vi "Error classifier.vi"(11 "Error in":errorcluster) -> (4 "Classified Ouput Error":T1, 15 "Error out":errorcluster)   [LabVIEW 2020, in "PSRR Monitor.lvlib"]
doc: "This VI is used to classify the error which is generated by the PSRR meter and will give the classified error to the main PSRR module."
uses:
  PSRR Monitor.lvlib
  Typedefs/Error Details.ctl
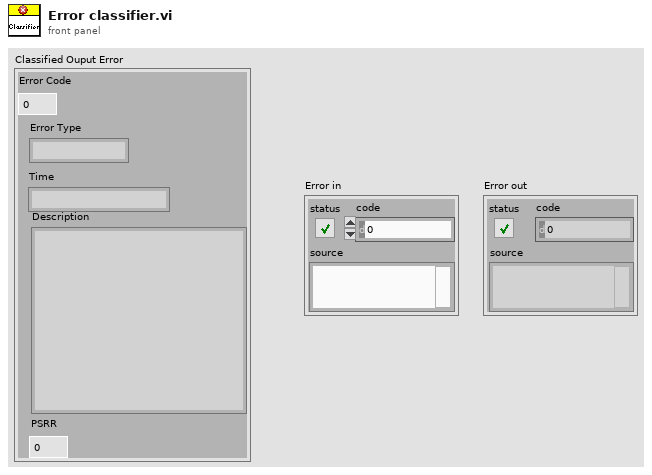
[diagram p1: front panel]
types:
  T1 = typedef "Error Details.ctl" = cluster{"Error Code":i32, "Error Type":string, "Time":string, "Description":string, "PSRR":i32}
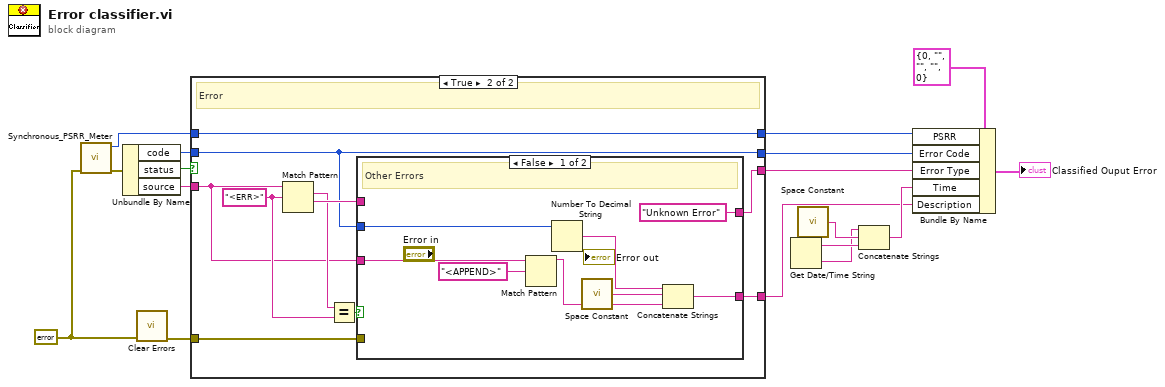
[diagram p0: block diagram]
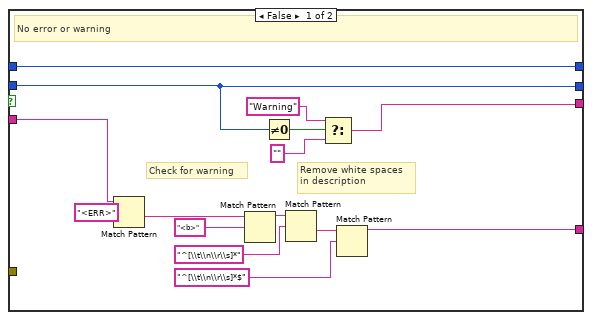
[diagram p2: hidden frame]
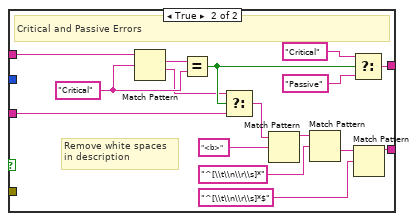
[diagram p3: hidden frame]
diagram:
  w2 = errorcluster {"status"=FALSE, "code"=0, "source"=""} ("error in")
  n1 = call "Synchronous_PSRR_Meter.vi"("error in"=w2) -> ("error out"=w17:errorcluster, "PSRR (dB)"=w4:i32)  [unwired: 9 in]
  n2 = Unbundle By Name(w17) -> ("code"=w14:i32, "status"=w15:bool, "source"=w16:string)
  n3 = call <vilib>:"Clear Errors.vi"("error in (no error)"=w2) -> ("error out"=w1:errorcluster)  [unwired: 5 in, 1 out]
  n4 = case shown="True" w15 {
    tunnel: w16 -> [w26 w36]
    tunnel: w14 -> [w29 w35]
    tunnel: [w29 w35] -> w12
    tunnel: [w28 w42] -> w11
    tunnel: [w19 w40] -> w5
    tunnel: w4 -> [w18 w34]
    tunnel: [w18 w34] -> w3
    tunnel: w1 -> [_ w33]
    frame False {
      # "Check for warning"
      # "Remove white spaces\nin description"
      # "No error or warning"
      n5 = Match Pattern(string=w26, regular expression="<ERR>") -> (after substring=w20:string)  [unwired: 1 in, 3 out]
      n6 = Match Pattern(string=w20, regular expression="<b>") -> (before substring=w21:string)  [unwired: 1 in, 3 out]
      n7 = Not Equal To 0?(x=w29) -> (x != 0?=w32:bool)
      n8 = Match Pattern(string=w21, regular expression="^[\\t\\n\\r\\s]*") -> (after substring=w25:string)  [unwired: 1 in, 3 out]
      n9 = Select(t="Warning", s=w32, f="") -> (s? t:f=w28:string)
      n10 = Match Pattern(string=w25, regular expression="^[\\t\\n\\r\\s]*$") -> (before substring=w19:string)  [unwired: 1 in, 3 out]
    }
    frame True {
      w37 = "<ERR>" ("regular expression")
      # "Error"
      n11 = Match Pattern(string=w36, regular expression=w37) -> (match substring=w38:string, after substring=w41:string)  [unwired: 1 in, 2 out]
      n12 = Equal?(x=w38, y=w37) -> (x = y?=w39:bool)
      n13 = case shown="False" w39 {
        tunnel: ["Unknown Error" ("regular expression") w63] -> w42
        tunnel: w41 -> [_ w59]
        tunnel: [w43 w52] -> w40
        tunnel: w36 -> [w49 w51]
        tunnel: w35 -> [w47 _]
        tunnel: w33 -> [_ _]
        frame False {
          # "Other Errors"
          n14 = Match Pattern(string=w49, regular expression="<APPEND>") -> (before substring=w45:string)  [unwired: 1 in, 3 out]
          n15 = Number To Decimal String(number=w47) -> (decimal integer string=w46:string)  [unwired: 1 in]
          n16 = call <vilib>:"Space Constant.vi"() -> ("String"=w44:string)
          n17 = Concatenate Strings(w46, w44, w45) -> (w43:string)
        }
        frame True {
          w65 = "Critical" ("regular expression")
          # "Remove white spaces\nin description"
          # "Critical and Passive Errors"
          n18 = Match Pattern(string=w59, regular expression=w65) -> (match substring=w66:string, after substring=w60:string)  [unwired: 1 in, 2 out]
          n19 = Equal?(x=w66, y=w65) -> (x = y?=w61:bool)
          n20 = Select(t=w60, s=w61, f=w51) -> (s? t:f=w53:string)
          n21 = Match Pattern(string=w53, regular expression="<b>") -> (before substring=w58:string)  [unwired: 1 in, 3 out]
          n22 = Match Pattern(string=w58, regular expression="^[\\t\\n\\r\\s]*") -> (after substring=w57:string)  [unwired: 1 in, 3 out]
          n23 = Select(t="Critical" ("regular expression"), s=w61, f="Passive") -> (s? t:f=w63:string)
          n24 = Match Pattern(string=w57, regular expression="^[\\t\\n\\r\\s]*$") -> (before substring=w52:string)  [unwired: 1 in, 3 out]
        }
      }
    }
  }
  n25 = Get Date/Time String() -> (date string=w9:string, time string=w8:string)  [unwired: 3 in]
  n26 = call <vilib>:"Space Constant.vi"() -> ("String"=w10:string)
  n27 = Concatenate Strings(w8, w10, w9) -> (w7:string)
  n28 = Bundle By Name(cluster=T1 {"Error Code"=0, "Error Type"="", "Time"="", "Description"="", "PSRR"=0}, "PSRR"=w3, "Error Code"=w12, "Error Type"=w11, "Time"=w7, "Description"=w5) -> (→"Classified Ouput Error":T1)
